vi "Write VarMessage.vi"(8 "error in (no error)":errorcluster, 9 "Varient":variant, 10 "Label":string) -> (0 "error out":errorcluster, 3 "Message":refnum<class "VarMessage.lvclass">)   [LabVIEW 2011, in "Messenging.lvlib" / "VarMessage.lvclass"]
uses:
  VarMessage/VarMessage.lvclass
  VarMessage/VarMessage.lvclass/VarMessage.ctl
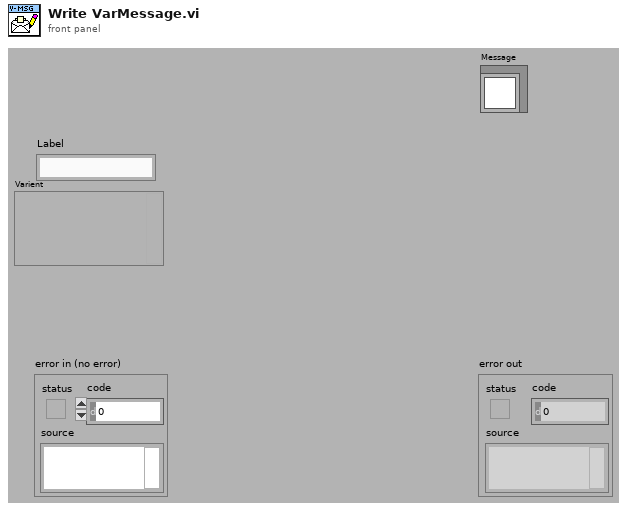
[diagram p1: front panel]
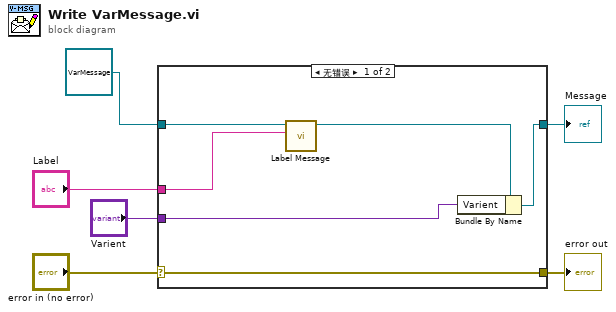
[diagram p0: block diagram]
diagram:
  n1 = case shown="无错误" "error in (no error)" {
    selector: "error in (no error)" -> [w12 w13]
    tunnel: [w12 w13] -> w5
    tunnel: [w11 w14] -> w4
    tunnel: refnum<class "VarMessage.lvclass"> refnum ("VarMessage.lvclass") -> [w9 w14]
    tunnel: "Label" -> [w8 _]
    tunnel: "Varient" -> [w10 _]
    frame No Error {
      n2 = call-dynamic "Label Message.vi"("Label"=w8, "Message"=w9) -> ("Message"=w7:refnum<class "VarMessage.lvclass">)  [unwired: 1 in, 8 out]
      n3 = Bundle By Name(cluster=w7, "Varient"=w10) -> (w11:refnum<class "VarMessage.lvclass">)
    }
    frame Error {
    }
  }
  "error out" <- w5
  "Message" <- w4
